vi "Write LoopScript.vi"(8 "error in (no error)":errorcluster, 10 "LoopScript":string[](array[string]), 11 "TestBase in":refnum<class "TestBase.lvclass">) -> (0 "error out":errorcluster, 3 "TestBase out":refnum<class "TestBase.lvclass">)   [LabVIEW 2014, in "TestBase.lvclass"]
uses:
  TestBase.lvclass
  TestBase.lvclass/TestBase.ctl
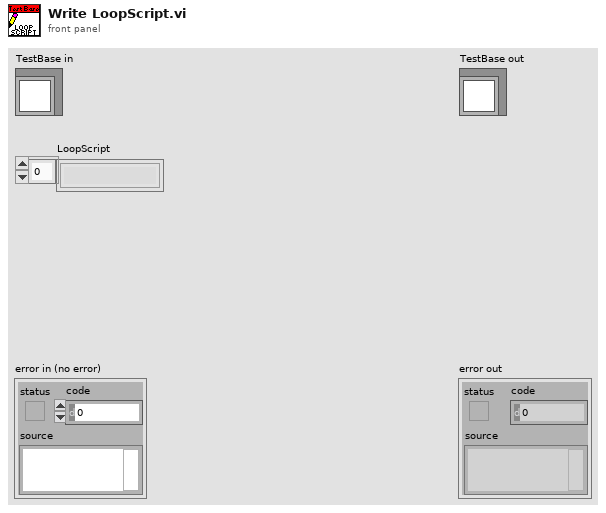
[diagram p1: front panel]
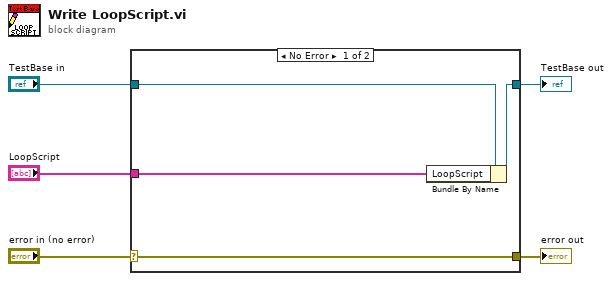
[diagram p0: block diagram]
diagram:
  n1 = case shown="No Error" "error in (no error)" {
    selector: "error in (no error)" -> [w9 w10]
    tunnel: [w9 w10] -> w4
    tunnel: [w7 w11] -> w2
    tunnel: "TestBase in" -> [w8 w11]
    tunnel: "LoopScript" -> [w6 _]
    frame No Error {
      n2 = Bundle By Name(cluster=w8, "LoopScript"=w6) -> (w7:refnum<class "TestBase.lvclass">)
    }
    frame Error {
    }
  }
  "error out" <- w4
  "TestBase out" <- w2
